vi "InitConstantsPerformReset.vi"   [LabVIEW 2019]
doc: "This VI sets constants and resets the global variables."
uses:
  constants.vi
  outputs.vi
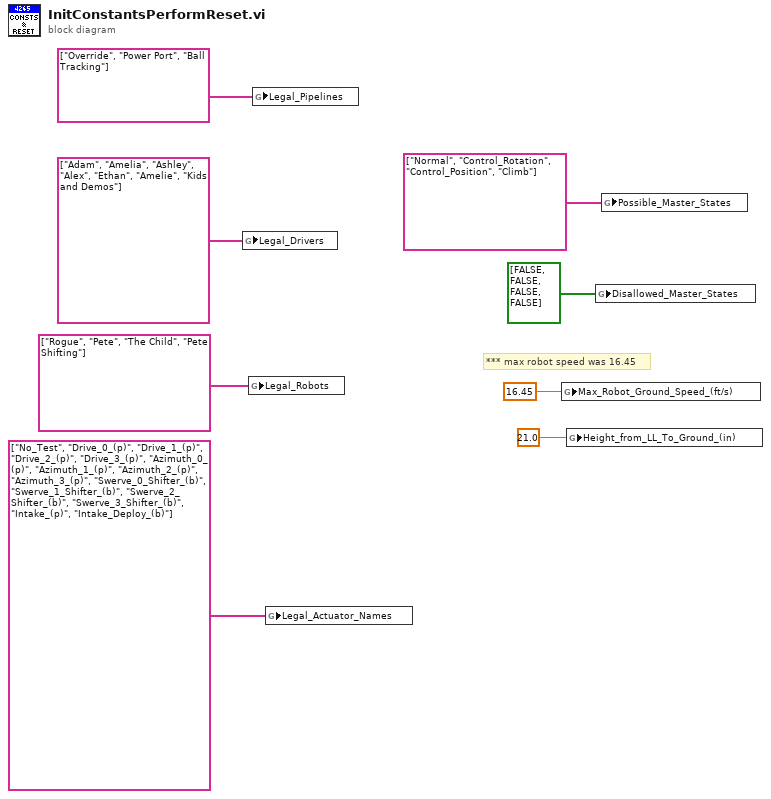
[diagram p0: block diagram]
diagram:
  # "*** max robot speed was 16.45"
  n1 = global write "constants.vi" "Legal_Drivers"(string[] ["Adam", "Amelia", "Ashley", "Alex", "Ethan", "Amelie", "Kids and Demos"] ("appended array")) -> ()
  n2 = global write "constants.vi" "Legal_Robots"(string[] ["Rogue", "Pete", "The Child", "Pete Shifting"] ("Legal_Actuator_Names")) -> ()
  n3 = global write "constants.vi" "Legal_Pipelines"(string[] ["Override", "Power Port", "Ball Tracking"] ("appended array")) -> ()
  n4 = global write "constants.vi" "Legal_Actuator_Names"(string[] ["No_Test", "Drive_0_(p)", "Drive_1_(p)", "Drive_2_(p)", "Drive_3_(p)", "Azimuth_0_(p)", "Azimuth_1_(p)", "Azimuth_2_(p)", "Azimuth_3_(p)", "Swerve_0_Shifter_(b)", "Swerve_1_Shifter_(b)", "Swerve_2_Shifter_(b)", "Swerve_3_Shifter_(b)", "Intake_(p)", "Intake_Deploy_(b)"] ("appended array")) -> ()
  n5 = global write "constants.vi" "Max_Robot_Ground_Speed_(ft/s)"(16.45 ("Max_Robot_Ground_Speed_(ft/s)")) -> ()
  n6 = global write "constants.vi" "Height_from_LL_To_Ground_(in)"(21.0 ("Max_Robot_Ground_Speed_(ft/s)")) -> ()
  n7 = global write "outputs.vi" "Disallowed_Master_States"(bool[] [FALSE, FALSE, FALSE, FALSE] ("appended array")) -> ()
  n8 = global write "constants.vi" "Possible_Master_States"(string[] ["Normal", "Control_Rotation", "Control_Position", "Climb"] ("appended array")) -> ()
